vi "07_DoRegression.vi"(9 "6 electrodes":bool, 10 "film H, nm":dbl=50.0, 11 "Input ChVoltage":T1) -> (0 "VoltageBelow, V":dbl, 2 "Regression":cluster{"VoltageRes, V":dbl, "Field, kV/cm":dbl}, 3 "PlotPoints":cluster{"Time":dbl[], "Voltage":dbl[]}(graph)={"Time"=[0.0, 0.00037111111108161925, 0.000510833333311085, 0.0006505555555405509, 0.0007766666666915019, 0.0009172222221968695, 0.0010569444444263353, 0.0011958333333152243, 0.0013350000000274223], "Voltage"=[5.89, 5.89, 5.89, 5.89, 5.89, 5.89, 5.89, 5.89, 5.89]})   [LabVIEW 2017]
uses:
  <vilib>/Analysis/6fits.llb/Curve Fitting Criteria.ctl
  <vilib>/Analysis/NI_AALPro.lvlib
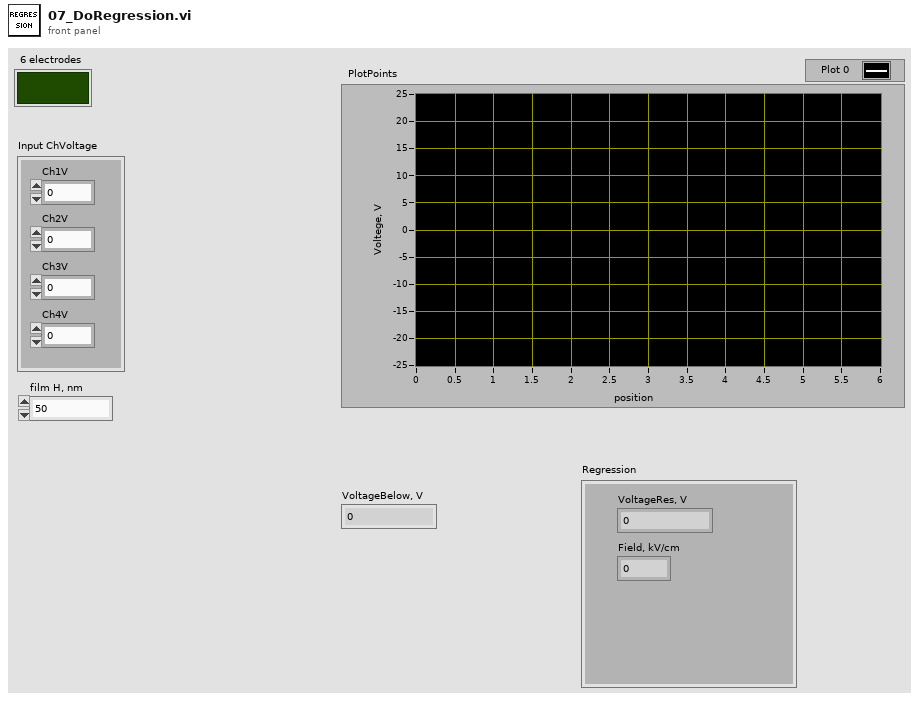
[diagram p1: front panel]
types:
  T1 = cluster{"Ch1V":dbl, "Ch2V":dbl, "Ch3V":dbl, "Ch4V":dbl}
  T2 = typedef "NI_AALPro.lvlib/Curve Fitting Criteria.ctl" = u16
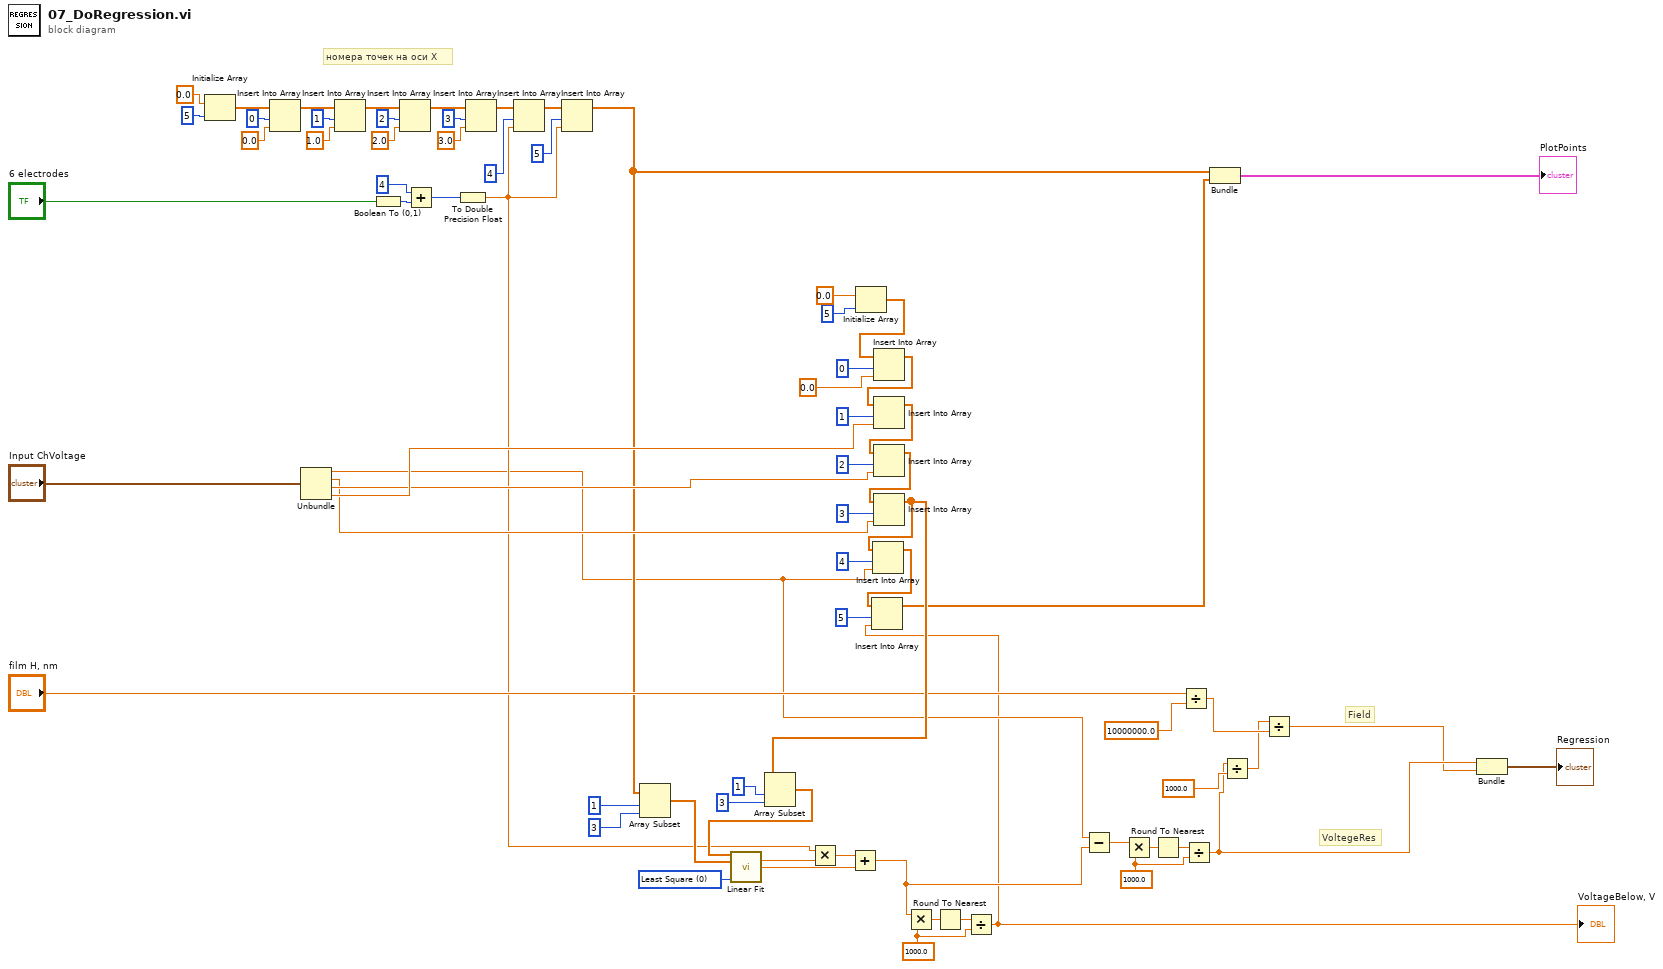
[diagram p0: block diagram]
diagram:
  w23 = 1000.0 ("y")
  w27 = 1000.0 ("y")
  w41 = T2 0 items=["Least Square", "Least Absolute Residual", "Bisquare"] ("method")
  # "Field"
  # "VoltegeRes"
  # "номера точек на оси X"
  n1 = Initialize Array(0.0 ("element"), 5 ("index")) -> (w61:dbl[])
  n2 = Insert Into Array(array=w61, index=0, new element=0.0 ("new element/subarray")) -> (w50:dbl[])
  n3 = Unbundle("Input ChVoltage") -> ("Ch1V"=w5:dbl, "Ch2V"=w9:dbl, "Ch3V"=w10:dbl, "Ch4V"=w11:dbl)
  n4 = Insert Into Array(array=w50, index=1, new element=1.0 ("new element/subarray")) -> (w49:dbl[])
  n5 = Boolean To (0,1)(Boolean="6 electrodes") -> (0, 1=w15:i16)
  n6 = Insert Into Array(array=w49, index=2, new element=2.0 ("new element/subarray")) -> (w48:dbl[])
  n7 = Add(x=i16 4, y=w15) -> (x+y=w13:i16)
  n8 = To Double Precision Float(number=w13) -> (double precision float=w8:dbl)
  n9 = Insert Into Array(array=w48, index=3, new element=3.0 ("new element/subarray")) -> (w37:dbl[])
  n10 = Insert Into Array(array=w37, index=4, new element=w8) -> (w47:dbl[])
  n11 = Insert Into Array(array=w47, index=5, new element=w8) -> (w7:dbl[])
  n12 = Array Subset(array=w7, index=1, length=3) -> (w36:dbl[])
  n13 = Initialize Array(0.0 ("element"), 5 ("dimension size")) -> (w64:dbl[])
  n14 = Insert Into Array(array=w64, index=0, new element=0.0 ("new element/subarray")) -> (w46:dbl[])
  n15 = Insert Into Array(array=w46, index=1, new element=w11) -> (w45:dbl[])
  n16 = Insert Into Array(array=w45, index=2, new element=w10) -> (w42:dbl[])
  n17 = Insert Into Array(array=w42, index=3, new element=w9) -> (w33:dbl[])
  n18 = Array Subset(array=w33, index=1, length=3) -> (w32:dbl[])
  n19 = call <vilib>:"Linear Fit.vi"("Y"=w32, "X"=w36, "method"=w41) -> ("slope"=w39:dbl, "intercept"=w40:dbl)  [unwired: 8 in, 3 out]
  n20 = Multiply(x=w8, y=w39) -> (x*y=w38:dbl)
  n21 = Add(x=w38, y=w40) -> (x+y=w22:dbl)
  n22 = Insert Into Array(array=w33, index=4, new element=w5) -> (w44:dbl[])
  n23 = Multiply(x=w22, y=w23) -> (x*y=w25:dbl)
  n24 = Round To Nearest(number=w25) -> (nearest integer value=w24:dbl)
  n25 = Divide(x=w24, y=w23) -> (x/y=w4:dbl)
  "VoltageBelow, V" <- w4
  n26 = Insert Into Array(array=w44, index=5, new element=w4) -> (w6:dbl[])
  n27 = Subtract(x=w5, y=w22) -> (x-y=w26:dbl)
  n28 = Multiply(x=w26, y=w27) -> (x*y=w29:dbl)
  n29 = Round To Nearest(number=w29) -> (nearest integer value=w28:dbl)
  n30 = Divide(x="film H, nm", y=10000000.0) -> (x/y=w18:dbl)
  n31 = Divide(x=w28, y=w27) -> (x/y=w2:dbl)
  n32 = Bundle(w7, w6) -> (→"PlotPoints":cluster{dbl[], dbl[]})  [unwired: 1 in]
  n33 = Divide(x=w2, y=1000.0) -> (x/y=w17:dbl)
  n34 = Divide(x=w17, y=w18) -> (x/y=w1:dbl)
  n35 = Bundle(w2, w1) -> (→"Regression":cluster{dbl, dbl})  [unwired: 1 in]
